vi "trash_Add Plugin Manager Error.vi"(8 "error in (no error)":errorcluster, 9 "String to Append":string, 10 "Error":T1, 11 "Insert Error":bool=TRUE) -> (0 "error out":errorcluster)   [LabVIEW 2021]
uses:
  CIFPluginManager.lvclass/CIFPluginManager.ctl
  <vilib>/CIF Foundation/CIF Utilities/Errors/Errors_CIF_U.lvlib
  typedef/trash_Errors.ctl
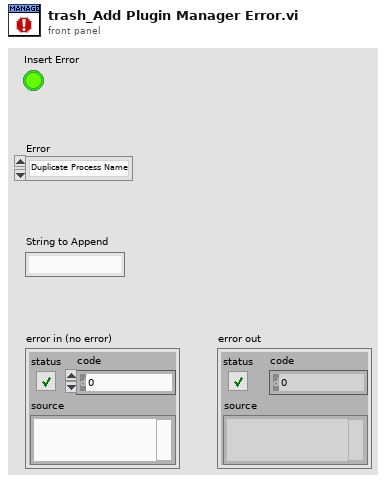
[diagram p1: front panel]
types:
  T1 = typedef "trash_Errors.ctl" = enum16{"Duplicate Process Name"}
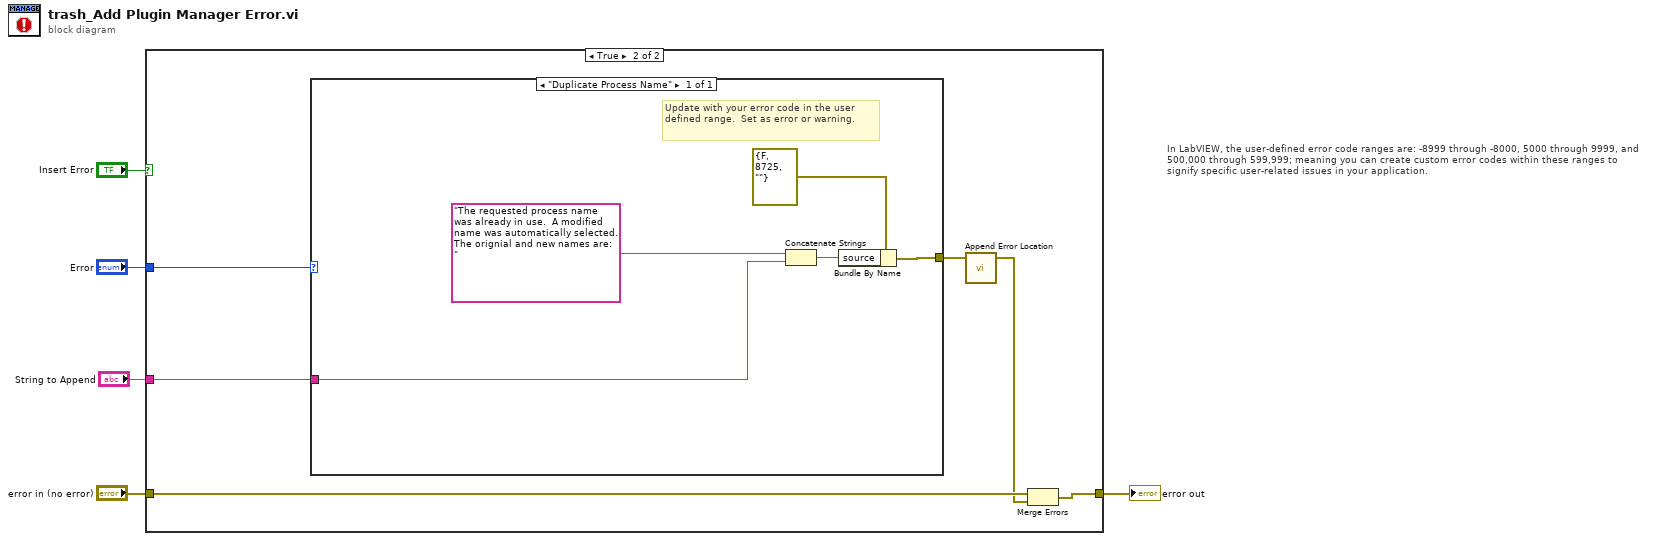
[diagram p0: block diagram]
diagram:
  # "In LabVIEW, the user-defined error code ranges are: -8999 through -8000, 5000 through 9999, and 500,000 through 599,999; meaning you can create custom error codes within these ranges to signify specific user-related issues in your application."
  n1 = case shown="True" "Insert Error" {
    tunnel: [w6 w9] -> w4
    tunnel: "error in (no error)" -> [w6 w10]
    tunnel: "Error" -> [_ w12]
    tunnel: "String to Append" -> [_ w11]
    frame False {
    }
    frame True {
      n2 = case shown="\"Duplicate Process Name\"" w12 {
        tunnel: w11 -> [w14]
        tunnel: [w16] -> w8
        frame "Duplicate Process Name" {
          # "Update with your error code in the user defined range.  Set as error or warning."
          n3 = Concatenate Strings("The requested process name was already in use.  A modified name was automatically selected.  The orignial and new names are: " ("source"), w14) -> (w13:string)
          n4 = Bundle By Name(cluster=errorcluster {"status"=FALSE, "code"=8725, "source"=""} ("Invalid ID"), "source"=w13) -> (w16:errorcluster)
        }
      }
      n5 = call <vilib>:"Append Error Location.vi"("error in (no error)"=w8) -> ("error out"=w7:errorcluster)  [unwired: 4 in]
      n6 = Merge Errors(w10, w7) -> (w9:errorcluster)
    }
  }
  "error out" <- w4
